vi "VL6180 Init.vi"(6 "Change Slave Address":u8=255 format="%02x", 8 "Error In":errorcluster, 9 "I2C Slave Address":u8=41 format="%x", 10 "I2C Channel":u8, 11 "LINX Resource":T1) -> (0 "Error Out":errorcluster, 2 "VL6180 Resource":T7 {"I2C Slave Address" format="%02x"}, 3 "LINX Resource":T1)   [LabVIEW 2018]
uses:
  VL6180X DEFS.ctl
  VL6180 Resource.ctl
  <vilib>/MakerHub/LINX/Private/Type Defs/Platform.ctl
  <vilib>/MakerHub/LINX/Private/Type Defs/Interface.ctl
  <vilib>/MakerHub/LINX/Private/Device/Type Defs/TCP Config.ctl
  <vilib>/MakerHub/LINX/Private/Device/Type Defs/Channels.ctl
  <vilib>/MakerHub/LINX/Private/Device/Type Defs/LINX Device Config.ctl
  <vilib>/MakerHub/LINX/Private/Type Defs/LINX Ref.ctl
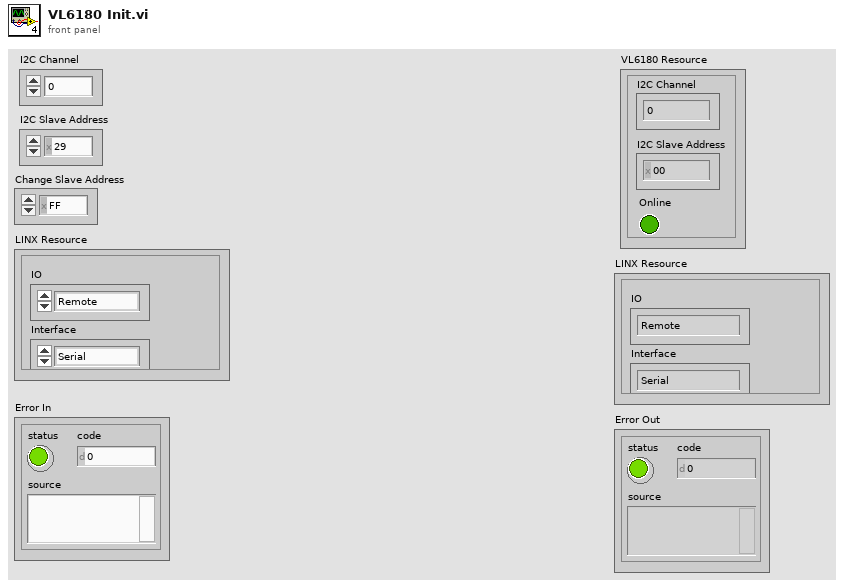
[diagram p1: front panel]
types:
  T1 = typedef "LMH-LINX.lvlib/LINX Ref.ctl" = cluster{"IO":T2, "Interface":T3, "LINX Device Config":T4}
  T2 = typedef "LMH-LINX.lvlib/Platform.ctl" = enum16{"Remote", "Local"}
  T3 = typedef "LMH-LINX.lvlib/Interface.ctl" = enum16{"Serial", "TCP"}
  T4 = typedef "LMH-LINX.lvlib/Device.lvlib/LINX Device Config.ctl" = cluster{"Interface":T3, "COM Port":refnum<visa-resource-name>, "TCP Configuration":T5, "Device Family":u8, "Device ID":u8, "Device Name":string, "TCP Ref":refnum<k5>, "Channels":T6}
  T5 = typedef "LMH-LINX.lvlib/Device.lvlib/TCP Config.ctl" = cluster{"IP Address":string, "Port":u16}
  T6 = typedef "LMH-LINX.lvlib/Channels.ctl" = cluster{"DI":u8[], "DO":u8[], "AI":u8[], "AO":u8[], "PWM":u8[], "QE":u8[], "UART":u8[], "I2C 2":u8[], "SPI":u8[], "CAN":u8[], "Servo":u8[], "AI Ref (V)":dbl, "AI Resolution (Bits)":u8, "AO Ref (V)":dbl, "AO Resolution (Bits)":u8}
  T7 = typedef "VL6180 Resource.ctl" = cluster{"I2C Channel":u8, "I2C Slave Address":u8, "Online":bool}
  T8 = typedef "VL6180X DEFS.ctl" = u16
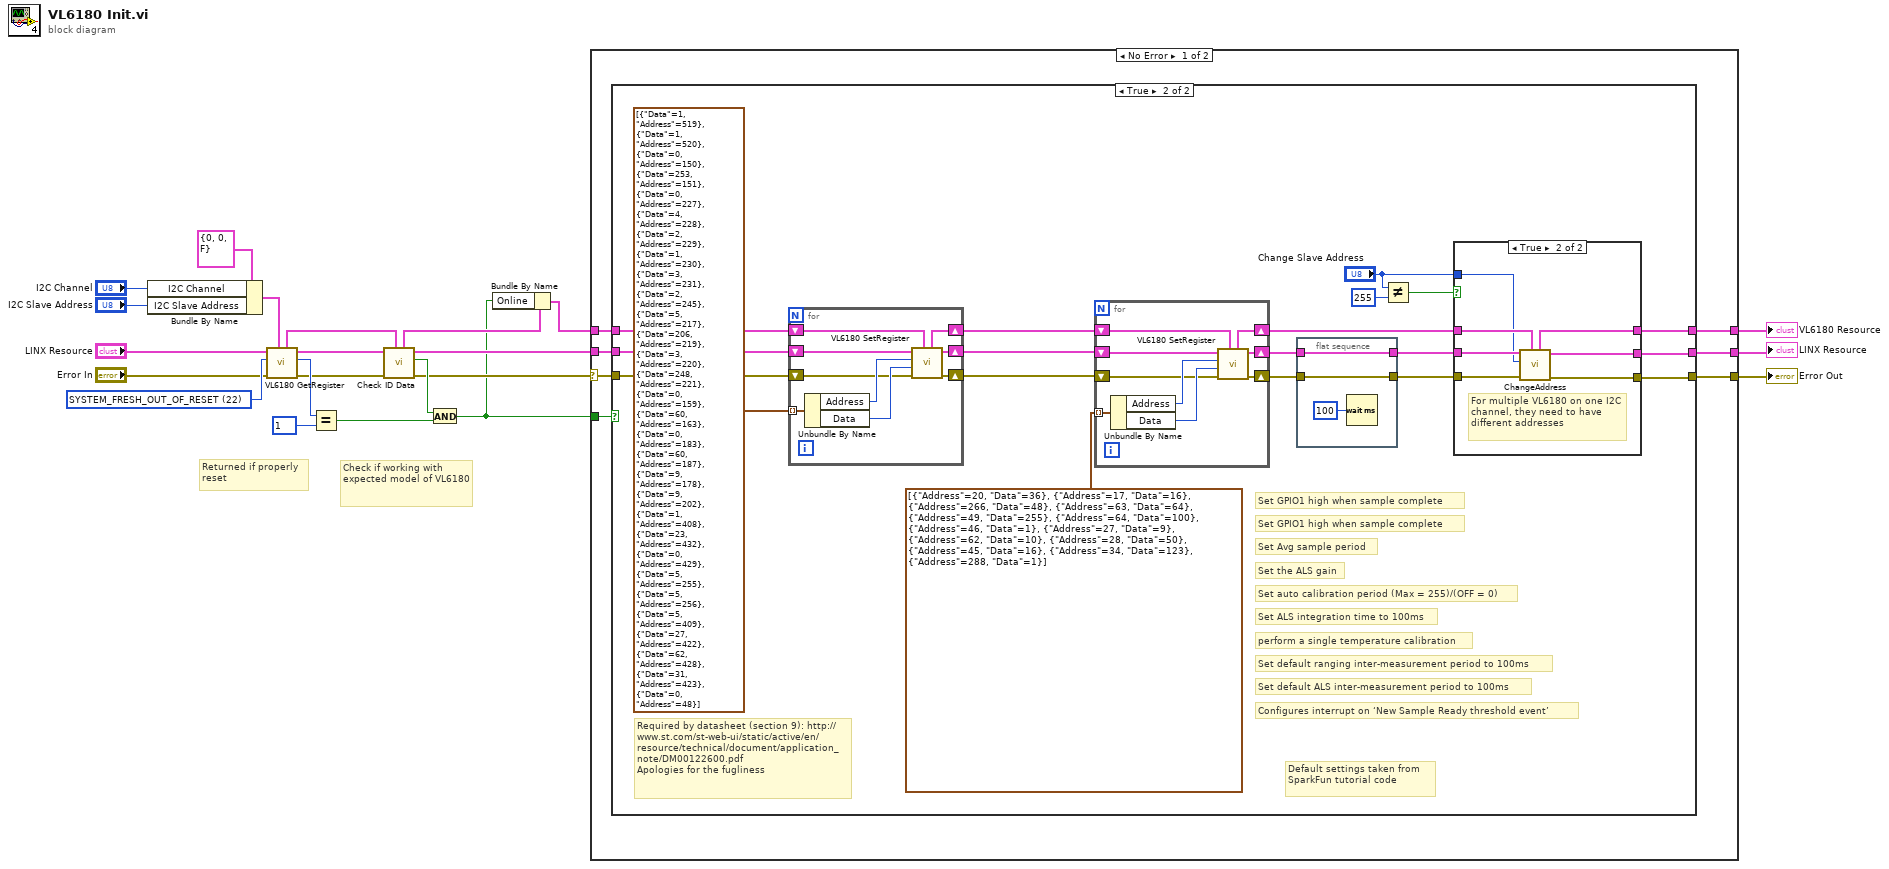
[diagram p0: block diagram]
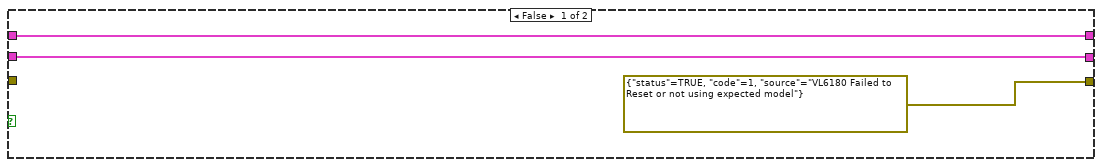
[diagram p2: hidden frame]
diagram:
  w20 = T8 22 items=["IDENTIFICATION_MODEL_ID"=0, "IDENTIFICATION_MODEL_REV_MAJOR"=1, "IDENTIFICATION_MODEL_REV_MINOR"=2, "IDENTIFICATION_MODULE_REV_MAJOR"=3, "IDENTIFICATION_MODULE_REV_MINOR"=4, "IDENTIFICATION_DATE"=6, "IDENTIFICATION_TIME"=8, "SYSTEM_MODE_GPIO0"=16, "SYSTEM_MODE_GPIO1"=17, "SYSTEM_HISTORY_CTRL"=18, "SYSTEM_INTERRUPT_CONFIG_GPIO"=20, "SYSTEM_INTERRUPT_CLEAR"=21, "SYSTEM_FRESH_OUT_OF_RESET"=22, "SYSTEM_GROUPED_PARAMETER_HOLD"=23, "SYSRANGE_START"=24, "SYSRANGE_THRESH_HIGH"=25, "SYSRANGE_THRESH_LOW"=26, "SYSRANGE_INTERMEASUREMENT_PERIOD"=27, "SYSRANGE_MAX_CONVERGENCE_TIME"=28, "SYSRANGE_CROSSTALK_COMPENSATION_RATE"=30, "SYSRANGE_CROSSTALK_VALID_HEIGHT"=33, "SYSRANGE_EARLY_CONVERGENCE_ESTIMATE"=34, "SYSRANGE_PART_TO_PART_RANGE_OFFSET"=36, "SYSRANGE_RANGE_IGNORE_VALID_HEIGHT"=37, "SYSRANGE_RANGE_IGNORE_THRESHOLD"=38, "SYSRANGE_MAX_AMBIENT_LEVEL_MULT"=44, "SYSRANGE_RANGE_CHECK_ENABLES"=45, "SYSRANGE_VHV_RECALIBRATE"=46, "SYSRANGE_VHV_REPEAT_RATE"=49, "SYSALS_START"=56, "SYSALS_THRESH_HIGH"=58, "SYSALS_THRESH_LOW"=60, "SYSALS_INTERMEASUREMENT_PERIOD"=62, "SYSALS_ANALOGUE_GAIN"=63, "SYSALS_INTEGRATION_PERIOD"=64, "RESULT_RANGE_STATUS"=77, "RESULT_ALS_STATUS"=78, "RESULT_INTERRUPT_STATUS_GPIO"=79, "RESULT_ALS_VAL"=80, "RESULT_HISTORY_BUFFER"=82, "RESULT_RANGE_VAL"=98, "RESULT_RANGE_RAW"=100, "RESULT_RANGE_RETURN_RATE"=102, "RESULT_RANGE_REFERENCE_RATE"=104, "RESULT_RANGE_RETURN_SIGNAL_COUNT"=108, "RESULT_RANGE_REFERENCE_SIGNAL_COUNT"=112, "RESULT_RANGE_RETURN_AMB_COUNT"=116, "RESULT_RANGE_REFERENCE_AMB_COUNT"=120, "RESULT_RANGE_RETURN_CONV_TIME"=124, "RESULT_RANGE_REFERENCE_CONV_TIME"=128, "READOUT_AVERAGING_SAMPLE_PERIOD"=266, "FIRMWARE_BOOTUP"=281, "FIRMWARE_RESULT_SCALER"=288, "I2C_SLAVE_DEVICE_ADDRESS"=530, "INTERLEAVED_MODE_ENABLE"=675] ("VL6180X Constants")
  # "Check if working with expected model of VL6180"
  # "Returned if properly\nreset"
  n1 = Bundle By Name(cluster=T7 {"I2C Channel"=0, "I2C Slave Address"=0, "Online"=FALSE} ("VL6180 Resource"), "I2C Channel"="I2C Channel", "I2C Slave Address"="I2C Slave Address") -> (w10:T7)
  n2 = call "VL6180 GetRegister.vi"("VL6180 Resource"=w10, "error in"="Error In", "VL6180X Constants"=w20, "LINX Resource"="LINX Resource") -> ("error out"=w15:errorcluster, "Data out"=w19:u8, "LINX Resource"=w9:T1, "VL6180 Resource"=w8:T7)  [unwired: 4 in]
  n3 = Equal?(x=w19, y=u8 1 ("Data 2")) -> (x = y?=w13:bool)
  n4 = call "Check ID Data.vi"("VL6180 Resource"=w8, "Error In"=w15, "LINX Resource"=w9) -> ("Error Out"=w11:errorcluster, "Same Model?"=w14:bool, "LINX Resource"=w16:T1, "VL6180 Resource"=w3:T7)  [unwired: 5 in]
  n5 = And(x=w14, y=w13) -> (x .and. y?=w2:bool)
  n6 = Bundle By Name(cluster=w3, "Online"=w2) -> (w1:T7)
  n7 = case shown="No Error" w11 {
    selector: w11 -> [w25 w84]
    tunnel: [w29 w84] -> w21
    tunnel: w16 -> [w28 w85]
    tunnel: [w27 w85] -> w7
    tunnel: w2 -> [w26 _]
    tunnel: w1 -> [w24 w83]
    tunnel: [w23 w83] -> w6
    frame No Error {
      n8 = case shown="True" w26 {
        tunnel: w25 -> [_ w49]
        tunnel: [errorcluster {"status"=TRUE, "code"=1, "source"="VL6180 Failed to Reset or not using expected model"} ("Error Out") w36] -> w29
        tunnel: w28 -> [w31 w51]
        tunnel: [w31 w37] -> w27
        tunnel: w24 -> [w30 w43]
        tunnel: [w30 w35] -> w23
        frame False {
        }
        frame True {
          # "Default settings taken from SparkFun tutorial code"
          # "Configures interrupt on ‘New Sample Ready threshold event’"
          # "Set default ALS inter-measurement period to 100ms"
          # "Set default ranging inter-measurement period to 100ms"
          # "perform a single temperature calibration"
          # "Set ALS integration time to 100ms"
          # "Set auto calibration period (Max = 255)/(OFF = 0)"
          # "Set the ALS gain"
          # "Set Avg sample period"
          # "Set GPIO1 high when sample complete"
          # "Set GPIO1 high when sample complete"
          # "Required by datasheet (section 9): http://www.st.com/st-web-ui/static/active/en/resource/technical/document/application_note/DM00122600.pdf\nApologies for the fugliness"
          n9 = for {
            tunnel: cluster{"Data":u8, "Address":u16}[] [{"Data"=1, "Address"=519}, {"Data"=1, "Address"=520}, {"Data"=0, "Address"=150}, {"Data"=253, "Address"=151}, {"Data"=0, "Address"=227}, {"Data"=4, "Address"=228}, {"Data"=2, "Address"=229}, {"Data"=1, "Address"=230}, {"Data"=3, "Address"=231}, {"Data"=2, "Address"=245}, {"Data"=5, "Address"=217}, {"Data"=206, "Address"=219}, {"Data"=3, "Address"=220}, {"Data"=248, "Address"=221}, {"Data"=0, "Address"=159}, {"Data"=60, "Address"=163}, {"Data"=0, "Address"=183}, {"Data"=60, "Address"=187}, {"Data"=9, "Address"=178}, {"Data"=9, "Address"=202}, {"Data"=1, "Address"=408}, {"Data"=23, "Address"=432}, {"Data"=0, "Address"=429}, {"Data"=5, "Address"=255}, {"Data"=5, "Address"=256}, {"Data"=5, "Address"=409}, {"Data"=27, "Address"=422}, {"Data"=62, "Address"=428}, {"Data"=31, "Address"=423}, {"Data"=0, "Address"=48}] -> [w81] mode=indexing
            shift-right: [w76] -> w46
            shift-left: w49 -> [w78]
            shift-right: [w77] -> w47
            shift-left: w51 -> [w82]
            shift-right: [w74] -> w42
            shift-left: w43 -> [w75]
            n10 = Unbundle By Name(w81) -> ("Address"=w80:u16, "Data"=w79:u8)
            n11 = call "VL6180 SetRegister.vi"("VL6180 Resource"=w75, "error in (no error)"=w78, "Data in"=w79, "Address"=w80, "LINX Resource"=w82) -> ("error out"=w76:errorcluster, "LINX Resource"=w77:T1, "VL6180 Resource"=w74:T7)  [unwired: 4 in]
          }
          n12 = for {
            tunnel: cluster{"Address":T8, "Data":u8}[] [{"Address"=20, "Data"=36}, {"Address"=17, "Data"=16}, {"Address"=266, "Data"=48}, {"Address"=63, "Data"=64}, {"Address"=49, "Data"=255}, {"Address"=64, "Data"=100}, {"Address"=46, "Data"=1}, {"Address"=27, "Data"=9}, {"Address"=62, "Data"=10}, {"Address"=28, "Data"=50}, {"Address"=45, "Data"=16}, {"Address"=34, "Data"=123}, {"Address"=288, "Data"=1}] -> [w72] mode=indexing
            shift-right: [w67] -> w44
            shift-left: w46 -> [w69]
            shift-right: [w68] -> w45
            shift-left: w47 -> [w73]
            shift-right: [w65] -> w38
            shift-left: w42 -> [w66]
            n13 = Unbundle By Name(w72) -> ("Address"=w71:T8, "Data"=w70:u8)
            n14 = call "VL6180 SetRegister.vi"("VL6180 Resource"=w66, "error in (no error)"=w69, "Data in"=w70, "Address"=w71, "LINX Resource"=w73) -> ("error out"=w67:errorcluster, "LINX Resource"=w68:T1, "VL6180 Resource"=w65:T7)  [unwired: 4 in]
          }
          n15 = flat-sequence {
            tunnel: w45 -> [w64]
            tunnel: w44 -> [w63]
            tunnel: [w64] -> w40
            tunnel: [w63] -> w39
            frame #0 {
              n16 = Wait (ms)(milliseconds to wait=u32 100) -> ()  [unwired: 1 out]
            }
          }
          n17 = Not Equal?(x="Change Slave Address", y=u8 255 ("Change Slave Address")) -> (x != y?=w34:bool)
          n18 = case shown="True" w34 {
            tunnel: w40 -> [w53 w61]
            tunnel: w39 -> [w52 w57]
            tunnel: w38 -> [w54 w60]
            tunnel: [w53 w59] -> w37
            tunnel: [w52 w58] -> w36
            tunnel: [w54 w56] -> w35
            tunnel: "Change Slave Address" -> [_ w55]
            frame False {
            }
            frame True {
              # "For multiple VL6180 on one I2C channel, they need to have different addresses"
              n19 = call "ChangeAddress.vi"("VL6180 Resource"=w60, "error in"=w57, "New Slave Address"=w55, "LINX Resource"=w61) -> ("error out"=w58:errorcluster, "LINX Resource"=w59:T1, "VL6180 Resource"=w56:T7)  [unwired: 5 in]
            }
          }
        }
      }
    }
    frame Error {
    }
  }
  "Error Out" <- w21
  "VL6180 Resource" <- w6
  "LINX Resource" <- w7
